vi "LinearFitPlot.vi"(8 "Y":dbl[](array[numeric]), 9 "Best Linear Fit":dbl[](array[numeric]), 10 "X":dbl[](array[numeric]), 11 "slope":dbl) -> ()   [LabVIEW 2020]
uses:
  <vilib>/Utility/file.llb/Write Delimited Spreadsheet (DBL).vi
panel:
  in  "Choose folder":path
  in  "Save to file":bool
  out "Attenuation[dB/cm]":dbl
  out "Spectras-Analiza":cluster{"X":dbl[], "Best Linear Fit":dbl[]}[](graph)
  in  "OK Button":bool
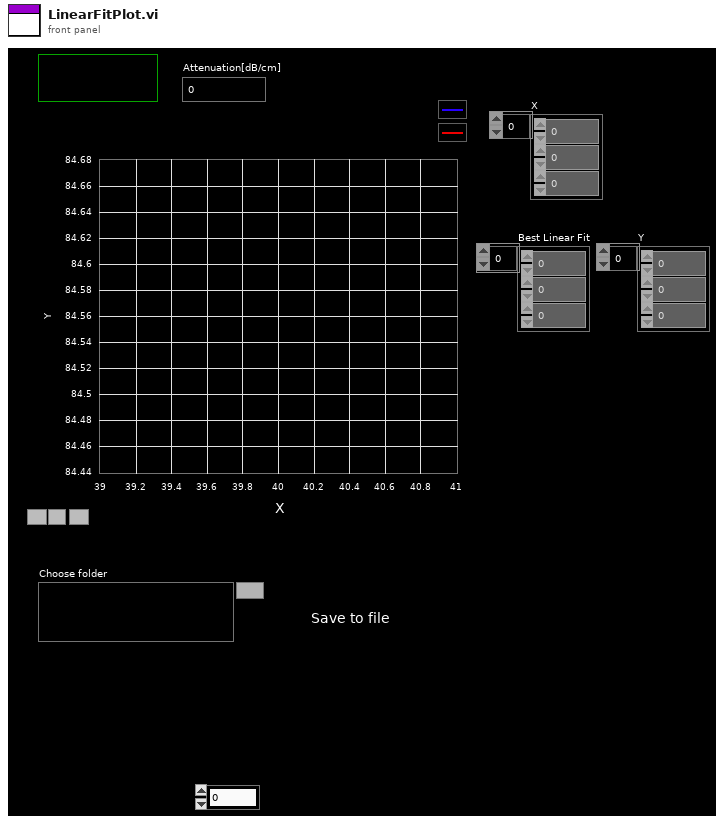
[diagram p1: front panel]
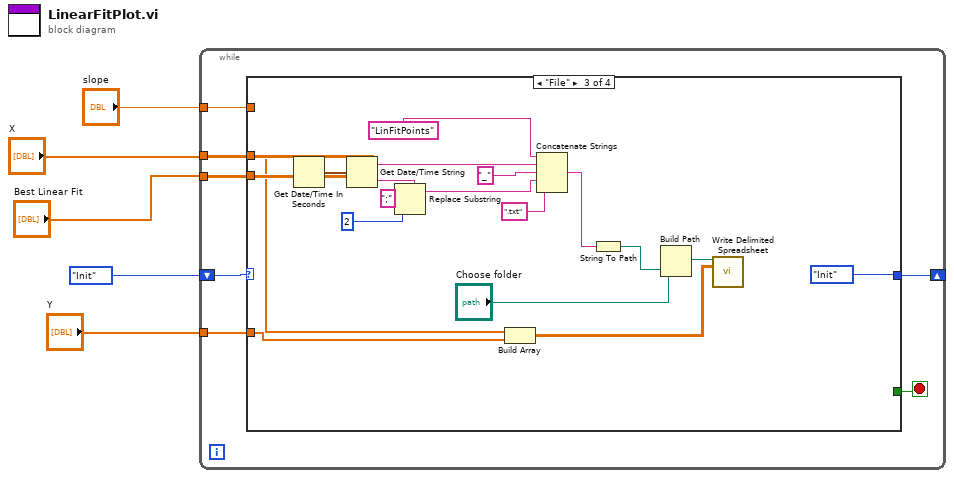
[diagram p0: block diagram]
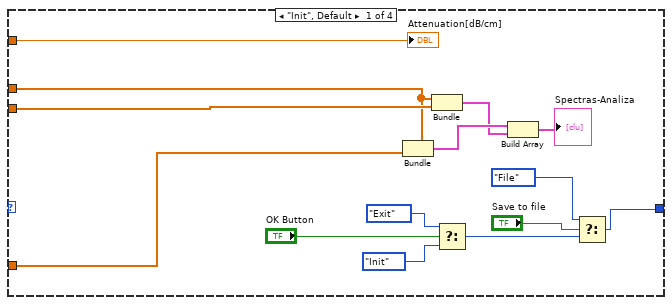
[diagram p2: hidden frame]
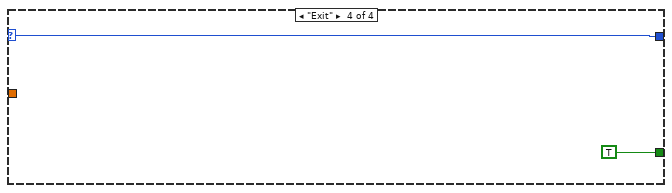
[diagram p4: hidden frame]
diagram:
  n1 = while {
    tunnel: "X" -> [w10]
    tunnel: "Best Linear Fit" -> [w12]
    tunnel: "slope" -> [w11]
    shift-right: [w7] -> _
    shift-left: enum16{"Init", "Wait", "File", "Exit"}."Init" -> [w9]
    tunnel: "Y" -> [w6]
    stop <- w8 stop-if-true
    n2 = case shown="\"File\"" w9 {
      selector: w9 -> [_ w27 _ w45]
      tunnel: w12 -> [w26 _ _ _]
      tunnel: w11 -> [w25 _ _ _]
      tunnel: w10 -> [w24 _ w30 _]
      tunnel: [_ _ _ TRUE] -> w8
      tunnel: [w16 w27 enum16{"Init", "Wait", "File", "Exit"}."Init" w45] -> w7
      tunnel: w6 -> [w13 _ w29 _]
      frame "Init", Default {
        n3 = Bundle("X"=w24, "Y"=w13) -> (w23:cluster{"X":dbl[], "Y":dbl[]})  [unwired: 1 in]
        n4 = Bundle("X"=w24, "Best Linear Fit"=w26) -> (w22:cluster{"X":dbl[], "Best Linear Fit":dbl[]})  [unwired: 1 in]
        n5 = Select(t=enum16{"Init", "Wait", "File", "Exit"}."Exit", s="OK Button", f=enum16{"Init", "Wait", "File", "Exit"}."Init") -> (s? t:f=w17:enum16{"Init", "Wait", "File", "Exit"})
        n6 = Build Array(w23, w22) -> (→"Spectras-Analiza":cluster{"X":dbl[], "Best Linear Fit":dbl[]}[])
        n7 = Select(t=enum16{"Init", "Wait", "File", "Exit"}."File", s="Save to file", f=w17) -> (s? t:f=w16:enum16{"Init", "Wait", "File", "Exit"})
        "Attenuation[dB/cm]" <- w25
      }
      frame "Wait" {
      }
      frame "File" {
        n8 = Get Date/Time In Seconds() -> (seconds since 1Jan1904=w43:timestamp)
        n9 = Get Date/Time String(seconds (now)=w43) -> (date string=w42:string, time string=w40:string)  [unwired: 2 in]
        n10 = Replace Substring(3:2 ("offset (0)"), 4:";" ("substring (\"\")"), 5:w40) -> (1:w36:string)  [unwired: 1 in, 1 out]
        n11 = Build Array(w30, w29) -> (w28:dbl[][])
        n12 = Concatenate Strings("LinFitPoints", w42, "_" ("string"), w36, ".txt" ("string")) -> (w34:string)
        n13 = String To Path(string=w34) -> (path=w31:path)
        n14 = Build Path(base path="Choose folder", name or relative path=w31) -> (appended path=w33:path)
        n15 = call-poly <vilib>:"Write Delimited Spreadsheet.vi"("file path (dialog if empty)"=w33, "2D data"=w28) -> ()  [unwired: 12 in, 2 out]
      }
      frame "Exit" {
      }
    }
  }
